vi "Cond Wait.vi"(8 "error in (no error)":errorcluster, 10 "Mutex in":T1, 11 "Cond in":T2) -> (0 "error out":errorcluster, 2 "Mutex out":T1, 3 "Cond out":T2)   [LabVIEW 2013, in "Linux RT IPC.POSIX Threads.lvlib" / "Cond.lvclass"]
doc: "Calls pthread_cond_timedwait() on the pthread cond object encapsulated by Cond.\n\nThis VI waits indefinitely for the conditional variable to be signaled. Ensure it is used in the correct ciscumstances to prevent encountering a deadlock.\n\nRefer to online POSIX documentation for more information."
uses:
  Cond.lvclass
  Controls/reference.ctl
  Mutex/Controls/reference.ctl
  Mutex/Mutex.lvclass
  POSIX Thread Object/POSIX Thread Object.lvclass/POSIX Thread Object.ctl
  POSIX Thread Object/Private VIs/libpthread path.vi
  POSIX Thread Object/Private VIs/get pthread error.vi
  POSIX Thread Object/POSIX Thread Object.lvclass
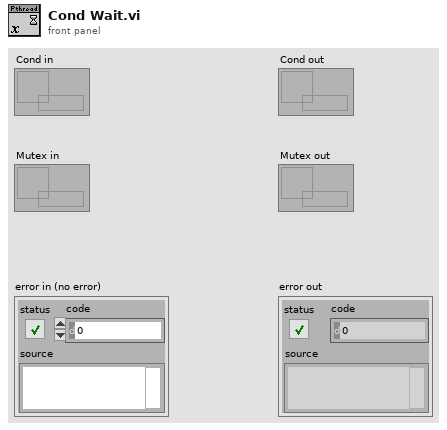
[diagram p1: front panel]
types:
  T1 = typedef "Linux RT IPC.POSIX Threads.lvlib/Mutex.lvclass/reference.ctl" = refnum<data-value>
  T2 = typedef "Linux RT IPC.POSIX Threads.lvlib/Cond.lvclass/reference.ctl" = refnum<data-value>
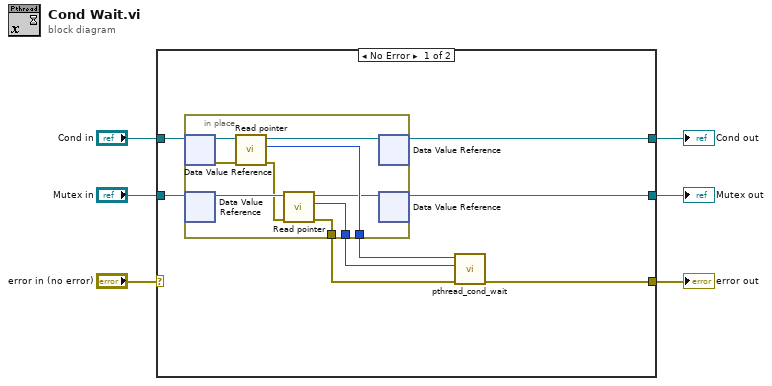
[diagram p0: block diagram]
diagram:
  n1 = case shown="No Error" "error in (no error)" {
    selector: "error in (no error)" -> [_ w26]
    tunnel: [w14 w26] -> w5
    tunnel: "Cond in" -> [w13 w25]
    tunnel: [w8 w25] -> w3
    tunnel: "Mutex in" -> [w12 w24]
    tunnel: [w7 w24] -> w1
    frame No Error {
      n2 = in-place {
        in-place-border: [w20] -> w9
        in-place-border: [w16] -> w11
        in-place-border: [w15] -> w10
        n3 = in-place-dvr #1(w13) -> (w23:refnum<class "Cond.lvclass">, w21:errorcluster)
        n4 = in-place-dvr #2(w12) -> (w19:refnum<class "Mutex.lvclass">)  [unwired: 1 out]
        n5 = call "Read pointer.vi"("error in (no error)"=w21, "POSIX Thread Object in"=w23) -> ("error out"=w17:errorcluster, "pointer"=w20:u64, "POSIX Thread Object out"=w22:refnum<class "Cond.lvclass">)  [unwired: 7 in]
        n6 = call "Read pointer.vi"("error in (no error)"=w17, "POSIX Thread Object in"=w19) -> ("error out"=w16:errorcluster, "pointer"=w15:u64, "POSIX Thread Object out"=w18:refnum<class "Mutex.lvclass">)  [unwired: 7 in]
        n7 = in-place-dvr #1(w22) -> (w8:T2)  [unwired: 1 out]
        n8 = in-place-dvr #2(w18) -> (w7:T1)  [unwired: 1 out]
      }
      n9 = call "pthread_cond_wait.vi"("error in (no error)"=w11, "mutex ptr in"=w10, "cond ptr in"=w9) -> ("error out"=w14:errorcluster)  [unwired: 6 in, 2 out]
    }
    frame Error {
    }
  }
  "Cond out" <- w3
  "error out" <- w5
  "Mutex out" <- w1
